vi "getGeneralLocation.vi"(8 "error in (no error)":errorcluster, 11 "RoundBuoy in":refnum<class "RoundBuoy.lvclass">) -> (0 "error out":errorcluster, 2 "General Location":T1 {"North" format="%#_10f"; "East" format="%#_8f"}, 3 "RoundBuoy out":refnum<class "RoundBuoy.lvclass">)   [LabVIEW 2011, in "RoundBuoy.lvclass"]
uses:
  RoundBuoy.lvclass
  2 Typedefs/UTM Location.ctl
  RoundBuoy.lvclass/RoundBuoy.ctl
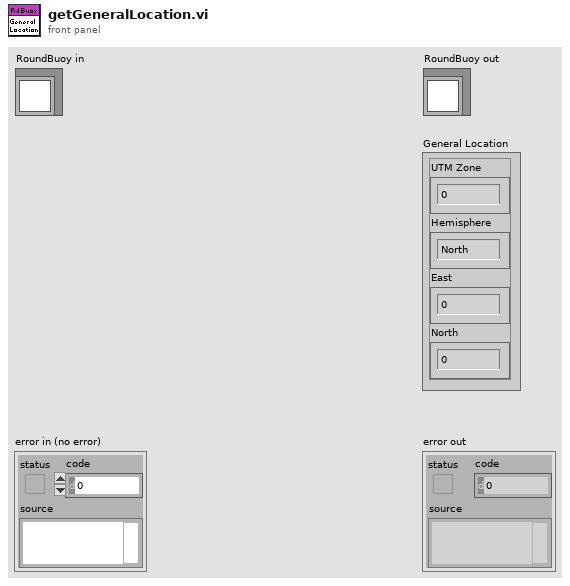
[diagram p1: front panel]
types:
  T1 = typedef "UTM Location.ctl" = cluster{"UTM Zone":dbl, "Hemisphere":enum16{"North", "South"}, "East":dbl, "North":dbl}
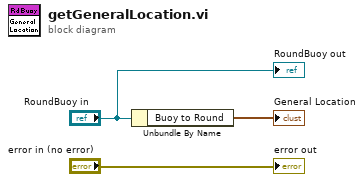
[diagram p0: block diagram]
diagram:
  n1 = Unbundle By Name("RoundBuoy in") -> ("Buoy to Round"=→"General Location":T1)
  "error out" <- "error in (no error)"
  "RoundBuoy out" <- "RoundBuoy in"
